vi "dfd_Convert CIC Params to String.vi"(6 "width (-)":i16, 7 "indent order":i32, 11 "CIC params":T1) -> (3 "string":string)   [LabVIEW 2017, in "NI_DigFilter_Process.lvlib"]
uses:
  <vilib>/addons/Digital Filter Design/NI_DigFilter_Process.lvlib
panel:
  out "filter type":enum16{"Lowpass", "Highpass"}(ring)
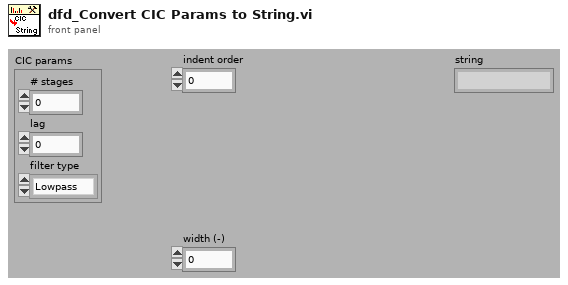
[diagram p1: front panel]
types:
  T1 = cluster{"# stages":i32, "lag":i32, "filter type":enum16{"Lowpass", "Highpass"}}
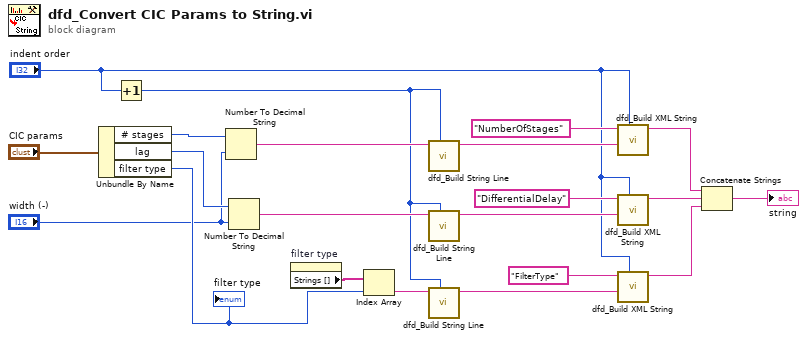
[diagram p0: block diagram]
diagram:
  n1 = Unbundle By Name("CIC params") -> ("# stages"=w18:i32, "lag"=w13:i32, "filter type"=w11:enum16{"Lowpass", "Highpass"})
  "filter type" <- w11
  n2 = Increment(x="indent order") -> (x+1=w7:i32)
  n3 = Number To Decimal String(number=w18, width (-)="width (-)") -> (decimal integer string=w19:string)
  n4 = Number To Decimal String(number=w13, width (-)="width (-)") -> (decimal integer string=w16:string)
  n5 = property on="filter type" class="Enum (strict)"() -> ("Strings []"=w12:string[])  [unwired: 2 in, 2 out]
  n6 = Index Array(array=w12, index=w11) -> (element=w10:string)
  n7 = call <vilib>:"dfd_Build String Line.vi"("indent order"=w7, "string"=w19) -> ("string line"=w20:string)  [unwired: 9 out]
  n8 = call <vilib>:"dfd_Build String Line.vi"("indent order"=w7, "string"=w16) -> ("string line"=w15:string)  [unwired: 9 out]
  n9 = call <vilib>:"dfd_Build String Line.vi"("indent order"=w7, "string"=w10) -> ("string line"=w8:string)  [unwired: 9 out]
  n10 = call <vilib>:"dfd_Build XML String.vi"("indent order"="indent order", "string in"=w20, "element name"="NumberOfStages") -> ("xml string out"=w5:string)  [unwired: 2 in, 6 out]
  n11 = call <vilib>:"dfd_Build XML String.vi"("indent order"="indent order", "string in"=w15, "element name"="DifferentialDelay") -> ("xml string out"=w4:string)  [unwired: 2 in, 6 out]
  n12 = call <vilib>:"dfd_Build XML String.vi"("indent order"="indent order", "string in"=w8, "element name"="FilterType") -> ("xml string out"=w3:string)  [unwired: 2 in, 6 out]
  n13 = Concatenate Strings(w5, w4, w3) -> (→"string":string)
